vi "UTIL EEG Filter Bank.vi"(8 "init/cont (init:F)":bool, 9 "Amplifier Gain":dbl(ring) items=["10X"=10.0, "100X"=100.0], 10 "Filter Coefficients from File":dbl[][](array[numeric]), 11 "EEG In":waveform(dbl)) -> (0 "Error Out":errorcluster, 2 "EEG Components":T1, 3 "Filtered EEG Out":waveform(dbl))   [LabVIEW 2017]
doc: "This VI applies a bank of BandPass Butterworth filters to the input EEG Waveform using an array of predetermined coefficients from MATLAB. It returns the Filtered EEG (0.5-45Hz) and a set of EEG components (Delta Low, Delta High, Theta, Alpha, Beta, Gamma, and Total). A notch filter at 60 Hz is also applied prior to the band filters.\n\nInputs:\n EEG In Waveform\n Error In\nOutputs:\n Filtered EEG Out Waveform\n EEG Components Cluster of Dbl, TYPE EEG Component\n Error Out"
uses:
  Types/TYPE EEG Components.ctl
  <vilib>/Analysis/baseanly.llb/Mean (DBL).vi
  <vilib>/Analysis/3filter.llb/IIR Filter (DBL).vi
  <vilib>/Analysis/NI_AALBase.lvlib
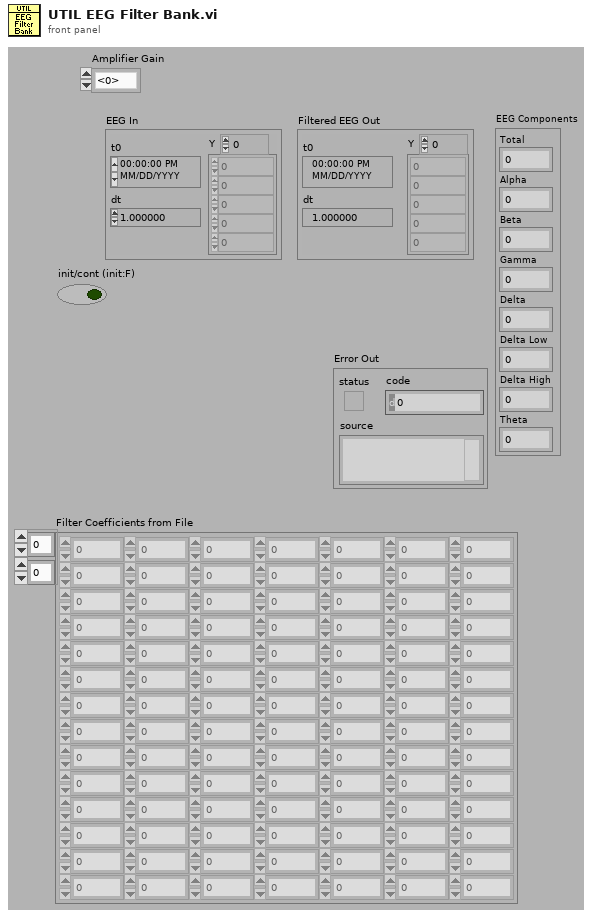
[diagram p1: front panel]
types:
  T1 = typedef "TYPE EEG Components.ctl" = cluster{"Total":dbl, "Alpha":dbl, "Beta":dbl, "Gamma":dbl, "Delta":dbl, "Delta Low":dbl, "Delta High":dbl, "Theta":dbl}
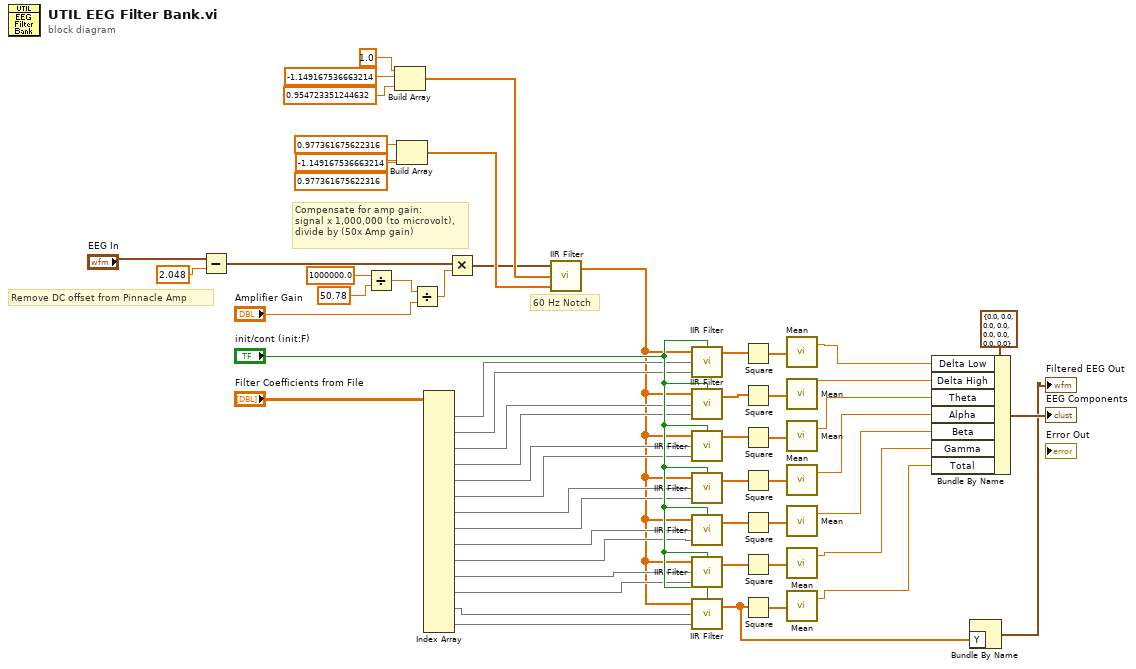
[diagram p0: block diagram]
diagram:
  # "Remove DC offset from Pinnacle Amp"
  # "60 Hz Notch"
  # "Compensate for amp gain:\nsignal x 1,000,000 (to microvolt), \ndivide by (50x Amp gain)"
  n1 = Subtract(x="EEG In", y=2.048) -> (x-y=w5:waveform(dbl))
  n2 = Divide(x=1000000.0, y=50.78) -> (x/y=w1:dbl)
  n3 = Build Array(1.0 ("element"), -1.149167536663214 ("element"), 0.954723351244632 ("element")) -> (w14:dbl[])
  n4 = Build Array(0.977361675622316 ("element"), -1.149167536663214 ("element"), 0.977361675622316 ("element")) -> (w13:dbl[])
  n5 = Divide(x=w1, y="Amplifier Gain") -> (x/y=w8:dbl)
  n6 = Index Array(array="Filter Coefficients from File") -> (element #1=w34:dbl[], element #2=w33:dbl[], element #3=w32:dbl[], element #4=w31:dbl[], element #5=w30:dbl[], element #6=w29:dbl[], element #7=w28:dbl[], element #8=w27:dbl[], element #9=w26:dbl[], element #10=w25:dbl[], element #11=w24:dbl[], element #12=w23:dbl[], element #13=w22:dbl[], element #14=w21:dbl[])  [unwired: 28 in]
  n7 = Multiply(x=w5, y=w8) -> (x*y=w9:waveform(dbl))
  n8 = call-poly <vilib>:"IIR Filter.vi"("Forward Coefficients"=w13, "Reverse Coefficients"=w14, "X"=w9) -> ("Filtered X"=w12:dbl[])  [unwired: 1 in, 1 out]
  n9 = call-poly <vilib>:"IIR Filter.vi"("init/cont (init:F)"="init/cont (init:F)", "Forward Coefficients"=w33, "Reverse Coefficients"=w34, "X"=w12) -> ("Filtered X"=w50:dbl[])  [unwired: 1 out]
  n10 = call-poly <vilib>:"IIR Filter.vi"("init/cont (init:F)"="init/cont (init:F)", "Forward Coefficients"=w31, "Reverse Coefficients"=w32, "X"=w12) -> ("Filtered X"=w51:dbl[])  [unwired: 1 out]
  n11 = call-poly <vilib>:"IIR Filter.vi"("init/cont (init:F)"="init/cont (init:F)", "Forward Coefficients"=w29, "Reverse Coefficients"=w30, "X"=w12) -> ("Filtered X"=w52:dbl[])  [unwired: 1 out]
  n12 = call-poly <vilib>:"IIR Filter.vi"("init/cont (init:F)"="init/cont (init:F)", "Forward Coefficients"=w27, "Reverse Coefficients"=w28, "X"=w12) -> ("Filtered X"=w53:dbl[])  [unwired: 1 out]
  n13 = call-poly <vilib>:"IIR Filter.vi"("init/cont (init:F)"="init/cont (init:F)", "Forward Coefficients"=w25, "Reverse Coefficients"=w26, "X"=w12) -> ("Filtered X"=w54:dbl[])  [unwired: 1 out]
  n14 = call-poly <vilib>:"IIR Filter.vi"("init/cont (init:F)"="init/cont (init:F)", "Forward Coefficients"=w23, "Reverse Coefficients"=w24, "X"=w12) -> ("Filtered X"=w55:dbl[])  [unwired: 1 out]
  n15 = call-poly <vilib>:"IIR Filter.vi"("init/cont (init:F)"="init/cont (init:F)", "Forward Coefficients"=w21, "Reverse Coefficients"=w22, "X"=w12) -> ("Filtered X"=w11:dbl[])  [unwired: 1 out]
  n16 = Square(x=w50) -> (x^2=w49:dbl[])
  n17 = Square(x=w51) -> (x^2=w48:dbl[])
  n18 = Square(x=w52) -> (x^2=w47:dbl[])
  n19 = Square(x=w53) -> (x^2=w46:dbl[])
  n20 = Square(x=w54) -> (x^2=w45:dbl[])
  n21 = Square(x=w55) -> (x^2=w44:dbl[])
  n22 = Square(x=w11) -> (x^2=w43:dbl[])
  n23 = call-poly <vilib>:"Mean.vi"("X"=w49) -> ("mean"=w42:dbl)  [unwired: 1 out]
  n24 = call-poly <vilib>:"Mean.vi"("X"=w48) -> ("mean"=w41:dbl)  [unwired: 1 out]
  n25 = call-poly <vilib>:"Mean.vi"("X"=w47) -> ("mean"=w40:dbl)  [unwired: 1 out]
  n26 = call-poly <vilib>:"Mean.vi"("X"=w46) -> ("mean"=w39:dbl)  [unwired: 1 out]
  n27 = call-poly <vilib>:"Mean.vi"("X"=w45) -> ("mean"=w38:dbl)  [unwired: 1 out]
  n28 = call-poly <vilib>:"Mean.vi"("X"=w44) -> ("mean"=w37:dbl)  [unwired: 1 out]
  n29 = call-poly <vilib>:"Mean.vi"("X"=w43) -> ("mean"=w36:dbl)  [unwired: 1 out]
  n30 = Bundle By Name(cluster=T1 {"Total"=0.0, "Alpha"=0.0, "Beta"=0.0, "Gamma"=0.0, "Delta"=0.0, "Delta Low"=0.0, "Delta High"=0.0, "Theta"=0.0} ("EEG Components"), "Delta Low"=w42, "Delta High"=w41, "Theta"=w40, "Alpha"=w39, "Beta"=w38, "Gamma"=w37, "Total"=w36) -> (→"EEG Components":T1)
  n31 = Bundle By Name("Y"=w11) -> (→"Filtered EEG Out":waveform(dbl))  [unwired: 1 in]
